vi "group Sync Write Change Param.vi"(6 "data_pos":u16, 7 "data_length":u16, 9 "data":u32, 10 "id":u8, 11 "group_num":i32) -> (3 "function return":u8)   [LabVIEW 2015, in "dxl_x86_c.lvlib"]
doc: "WINDECLSPEC uint8_t groupSyncWriteChangeParam (int group_num, uint8_t id, uint32_t data, uint16_t data_length, uint16_t data_pos);"
uses:
  dxl_x86_c.lvlib
  dxl_x86_c.dll
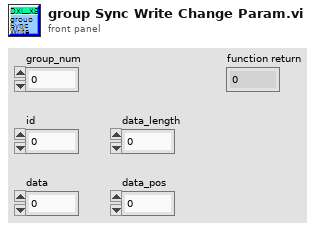
[diagram p1: front panel]
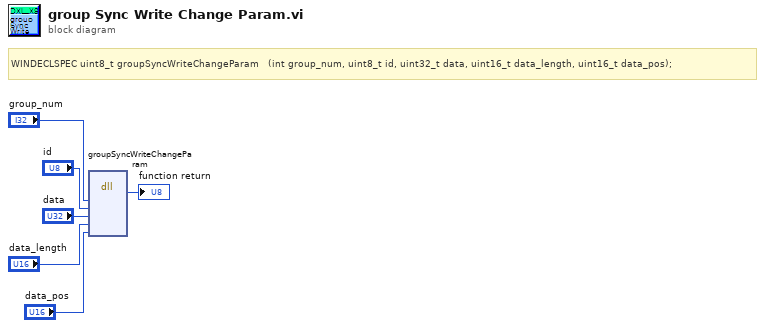
[diagram p0: block diagram]
diagram:
  # "WINDECLSPEC uint8_t groupSyncWriteChangeParam   (int group_num, uint8_t id, uint32_t data, uint16_t data_length, uint16_t data_pos);"
  n1 = dll-call lib="C:/Users/Platform/Desktop/LabVIEW/dxl_x86_c.lvlib/dxl_x86_c.*" fn="groupSyncWriteChangeParam"("group_num"="group_num", "id"="id", "data"="data", "data_length"="data_length", "data_pos"="data_pos") -> (→"function return":u8)  [unwired: 8 in, 2 out]
